vi "Output channel build.vi"(9 "Channel No":i32, 10 "DO":T1) -> (3 "Output channel":refnum<notifier>)   [LabVIEW 2020]
uses:
  Digital out put.ctl
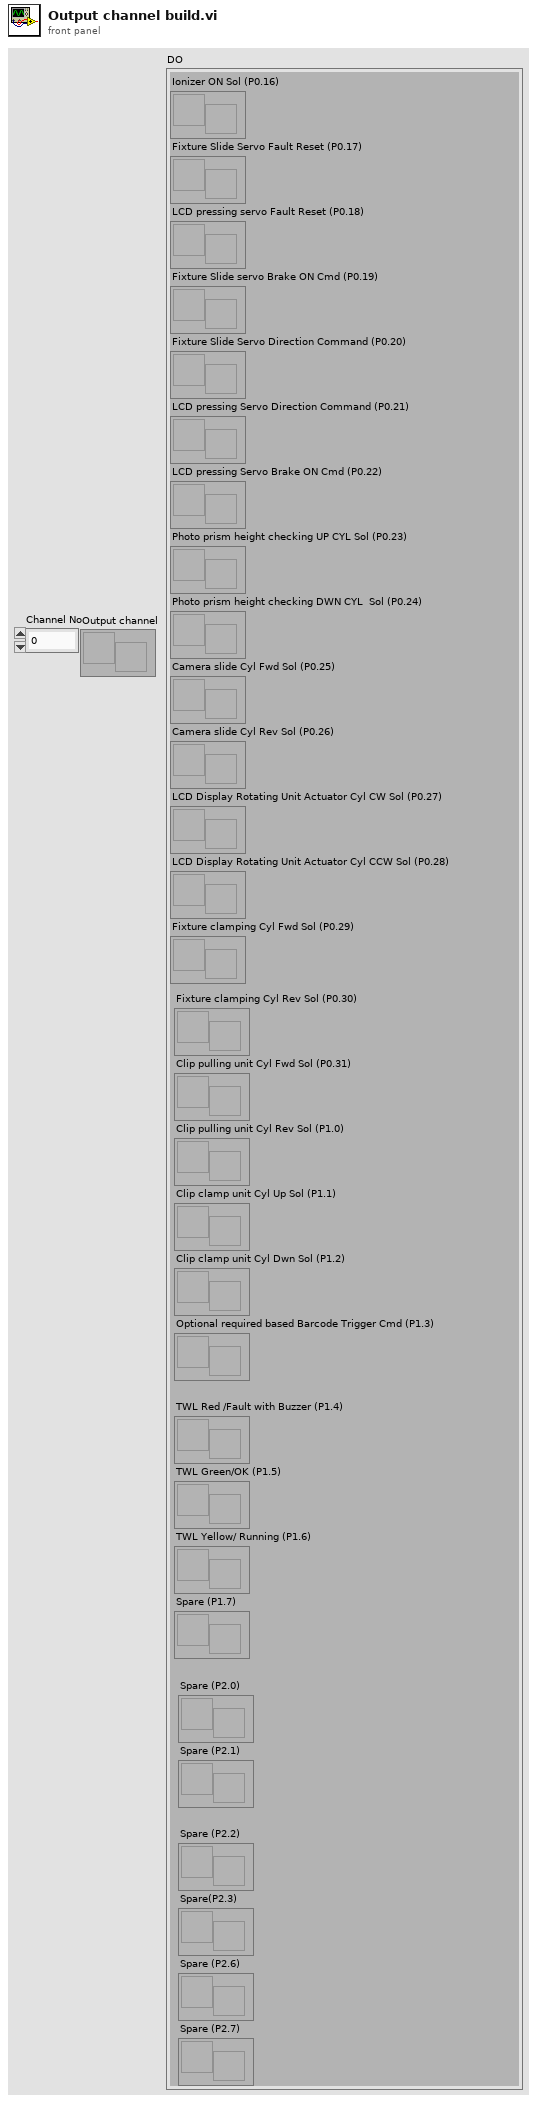
[diagram p1: front panel]
types:
  T1 = typedef "Digital out put.ctl" = cluster{"Ionizer ON Sol (P0.16)":refnum<notifier>, "Fixture Slide Servo Fault Reset (P0.17)":refnum<notifier>, "LCD pressing servo Fault Reset (P0.18)":refnum<notifier>, "Fixture Slide servo Brake ON Cmd (P0.19)":refnum<notifier>, "Fixture Slide Servo Direction Command (P0.20)":refnum<notifier>, "LCD pressing Servo Direction Command (P0.21)":refnum<notifier>, "LCD pressing Servo Brake ON Cmd (P0.22)":refnum<notifier>, "Photo prism height checking UP CYL Sol (P0.23)":refnum<notifier>, "Photo prism height checking DWN CYL  Sol (P0.24)":refnum<notifier>, "Camera slide Cyl Fwd Sol (P0.25)":refnum<notifier>, "Camera slide Cyl Rev Sol (P0.26)":refnum<notifier>, "LCD Display Rotating Unit Actuator Cyl CW Sol (P0.27)":refnum<notifier>, "LCD Display Rotating Unit Actuator Cyl CCW Sol (P0.28)":refnum<notifier>, "Fixture clamping Cyl Fwd Sol (P0.29)":refnum<notifier>, "Fixture clamping Cyl Rev Sol (P0.30)":refnum<notifier>, "Clip pulling unit Cyl Fwd Sol (P0.31)":refnum<notifier>, "Clip pulling unit Cyl Rev Sol (P1.0)":refnum<notifier>, "Clip clamp unit Cyl Up Sol (P1.1)":refnum<notifier>, "Clip clamp unit Cyl Dwn Sol (P1.2)":refnum<notifier>, "Optional required based Barcode Trigger Cmd (P1.3)":refnum<notifier>, "TWL Red /Fault with Buzzer (P1.4)":refnum<notifier>, "TWL Green/OK (P1.5)":refnum<notifier>, "TWL Yellow/ Running (P1.6)":refnum<notifier>, "Spare (P1.7)":refnum<notifier>, "Spare (P2.0)":refnum<notifier>, "Spare (P2.1)":refnum<notifier>, "Spare (P2.2)":refnum<notifier>, "Spare(P2.3)":refnum<notifier>, "Spare (P2.6)":refnum<notifier>, "Spare (P2.7) ":refnum<notifier>}
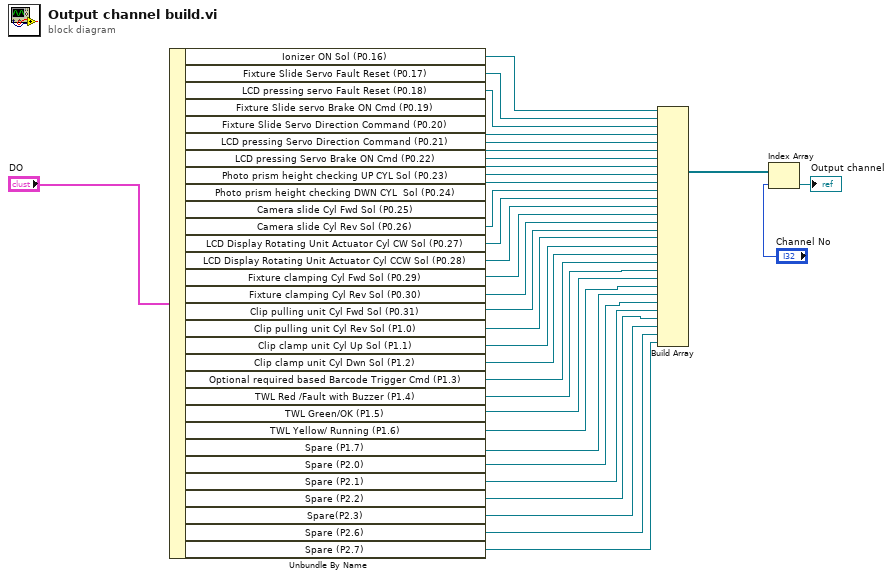
[diagram p0: block diagram]
diagram:
  n1 = Unbundle By Name("DO") -> ("Ionizer ON Sol (P0.16)"=w22:refnum<notifier>, "Fixture Slide Servo Fault Reset (P0.17)"=w23:refnum<notifier>, "LCD pressing servo Fault Reset (P0.18)"=w24:refnum<notifier>, "Fixture Slide servo Brake ON Cmd (P0.19)"=w25:refnum<notifier>, "Fixture Slide Servo Direction Command (P0.20)"=w26:refnum<notifier>, "LCD pressing Servo Direction Command (P0.21)"=w27:refnum<notifier>, "LCD pressing Servo Brake ON Cmd (P0.22)"=w28:refnum<notifier>, "Photo prism height checking UP CYL Sol (P0.23)"=w29:refnum<notifier>, "Photo prism height checking DWN CYL  Sol (P0.24)"=w30:refnum<notifier>, "Camera slide Cyl Fwd Sol (P0.25)"=w31:refnum<notifier>, "Camera slide Cyl Rev Sol (P0.26)"=w32:refnum<notifier>, "LCD Display Rotating Unit Actuator Cyl CW Sol (P0.27)"=w33:refnum<notifier>, "LCD Display Rotating Unit Actuator Cyl CCW Sol (P0.28)"=w34:refnum<notifier>, "Fixture clamping Cyl Fwd Sol (P0.29)"=w17:refnum<notifier>, "Fixture clamping Cyl Rev Sol (P0.30)"=w16:refnum<notifier>, "Clip pulling unit Cyl Fwd Sol (P0.31)"=w15:refnum<notifier>, "Clip pulling unit Cyl Rev Sol (P1.0)"=w14:refnum<notifier>, "Clip clamp unit Cyl Up Sol (P1.1)"=w13:refnum<notifier>, "Clip clamp unit Cyl Dwn Sol (P1.2)"=w12:refnum<notifier>, "Optional required based Barcode Trigger Cmd (P1.3)"=w11:refnum<notifier>, "TWL Red /Fault with Buzzer (P1.4)"=w10:refnum<notifier>, "TWL Green/OK (P1.5)"=w9:refnum<notifier>, "TWL Yellow/ Running (P1.6)"=w8:refnum<notifier>, "Spare (P1.7)"=w7:refnum<notifier>, "Spare (P2.0)"=w6:refnum<notifier>, "Spare (P2.1)"=w5:refnum<notifier>, "Spare (P2.2)"=w4:refnum<notifier>, "Spare(P2.3)"=w3:refnum<notifier>, "Spare (P2.6)"=w2:refnum<notifier>, "Spare (P2.7)"=w1:refnum<notifier>)
  n2 = Build Array(w22, w23, w24, w25, w26, w27, w28, w29, w30, w31, w32, w33, w34, w17, w16, w15, w14, w13, w12, w11, w10, w9, w8, w7, w6, w5, w4, w3, w2, w1) -> (w21:refnum<notifier>[])
  n3 = Index Array(array=w21, index="Channel No") -> (element=→"Output channel":refnum<notifier>)
